vi "tdms folder.vi"() -> ()   [LabVIEW 2019]
uses:
  DataSaver_class/DataSaver.lvclass
panel:
  out "dup path":path
  out "selected path":path
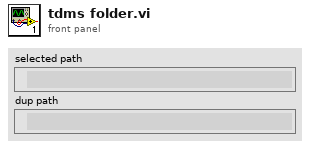
[diagram p1: front panel]
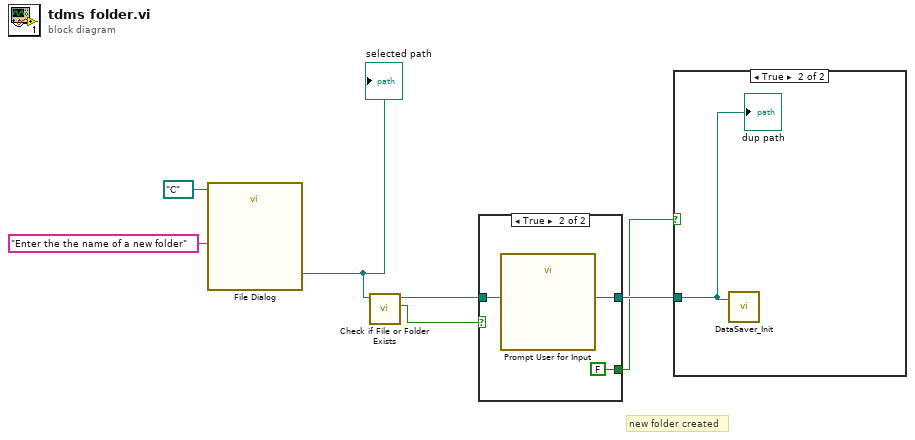
[diagram p0: block diagram]
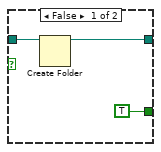
[diagram p3: hidden frame]
diagram:
  # "new folder created"
  n1 = call "File Dialog"("start path"=path "C:/", "prompt"="Enter the the name of a new folder") -> ("selected path"=w5:path)  [unwired: 10 in, 3 out]
  "selected path" <- w5
  n2 = call <vilib>:"Check if File or Folder Exists.vi"("path"=w5) -> ("file or folder exists?"=w3:bool, "dup path"=w4:path)  [unwired: 8 in, 1 out]
  n3 = case shown="True" w3 {
    tunnel: [w10 w12] -> w7
    tunnel: w4 -> [w9 w12]
    tunnel: [TRUE FALSE] -> w1
    frame False {
      n4 = Create Folder(path (use dialog)=w9) -> (created path=w10:path)  [unwired: 2 in, 2 out]
    }
    frame True {
      n5 = call "Prompt User for Input"() -> ()  [unwired: 18 in, 2 out]
    }
  }
  n6 = case shown="True" w1 {
    tunnel: w7 -> [_ w13]
    frame False {
    }
    frame True {
      n7 = call "DataSaver_Init.vi"("FolderPath"=w13) -> ()  [unwired: 17 in, 2 out]
      "dup path" <- w13
    }
  }
